vi "IMUread.vi"() -> ()   [LabVIEW 2015]
doc: "The myRIO Project template acquires acceleration data from the onboard accelerometer and displays the changes of acceleration values in a waveform chart."
uses:
  <vilib>/myRIO/Instrument Drivers/Onboard IO/I2C/typedefs/I2C User Configuration.ctl
  <vilib>/myRIO/Instrument Drivers/Onboard IO/I2C/typedefs/I2C Transfer Rate.ctl
  <vilib>/Platform/TimedLoop/XDataNode/timing_clust.ctl
  <vilib>/Platform/TimedLoop/XDataNode/nitl_modes.ctl
  <vilib>/Platform/TimedLoop/XDataNode/wakeup.ctl
  <vilib>/myRIO/Common/Instrument Driver Framework/myRIO v1.0/UART/vis/myRIO v1.0 Close UART.vi
  <vilib>/Utility/error.llb/Error Cluster From Error Code.vi
  <vilib>/myRIO/Common/Instrument Driver Framework/myRIO v1.0/I2C/vis/myRIO v1.0 Configure I2C.vi
  <vilib>/myRIO/Common/Instrument Driver Framework/myRIO v1.0/I2C/vis/myRIO v1.0 Write I2C.vi
  <vilib>/myRIO/Common/Instrument Driver Framework/myRIO v1.0/I2C/vis/myRIO v1.0 Read I2C.vi
  <vilib>/myRIO/Common/Instrument Driver Framework/Utilities/vis/FPGA Ref Manager.vi
  <vilib>/myRIO/Common/Instrument Driver Framework/myRIO v1.0/myRIO v1.0 Reset FPGA.vi
  <vilib>/myRIO/Common/Instrument Driver Framework/myRIO v1.0/IRQ/vis/myRIO v1.0 IRQ Info FGV.vi
  <vilib>/myRIO/Common/Instrument Driver Framework/myRIO v1.0/IRQ/vis/myRIO v1.0 Timer IRQ Info FGV.vi
  <vilib>/myRIO/Common/Instrument Driver Framework/myRIO v1.0/IRQ/vis/myRIO v1.0 ISR Agent.vi
  <vilib>/platform/TimedLoop/XDataNode/XDataNode.xnode
  <vilib>/myRIO/Instrument Drivers/Utilities/Utilities.lvlib
  <vilib>/myRIO/Instrument Drivers/Onboard IO/I2C/I2C.lvlib
  <vilib>/Platform/TimedLoop/XDataNode/XDNodeRunTimeDep.lvlib
panel:
  out "Mag Chart":cluster{dbl, dbl, dbl}(graph)
  out "Acc Chart":cluster{dbl, dbl, dbl}(graph)
  out "Gyro Chart":cluster{dbl, dbl, dbl}(graph)
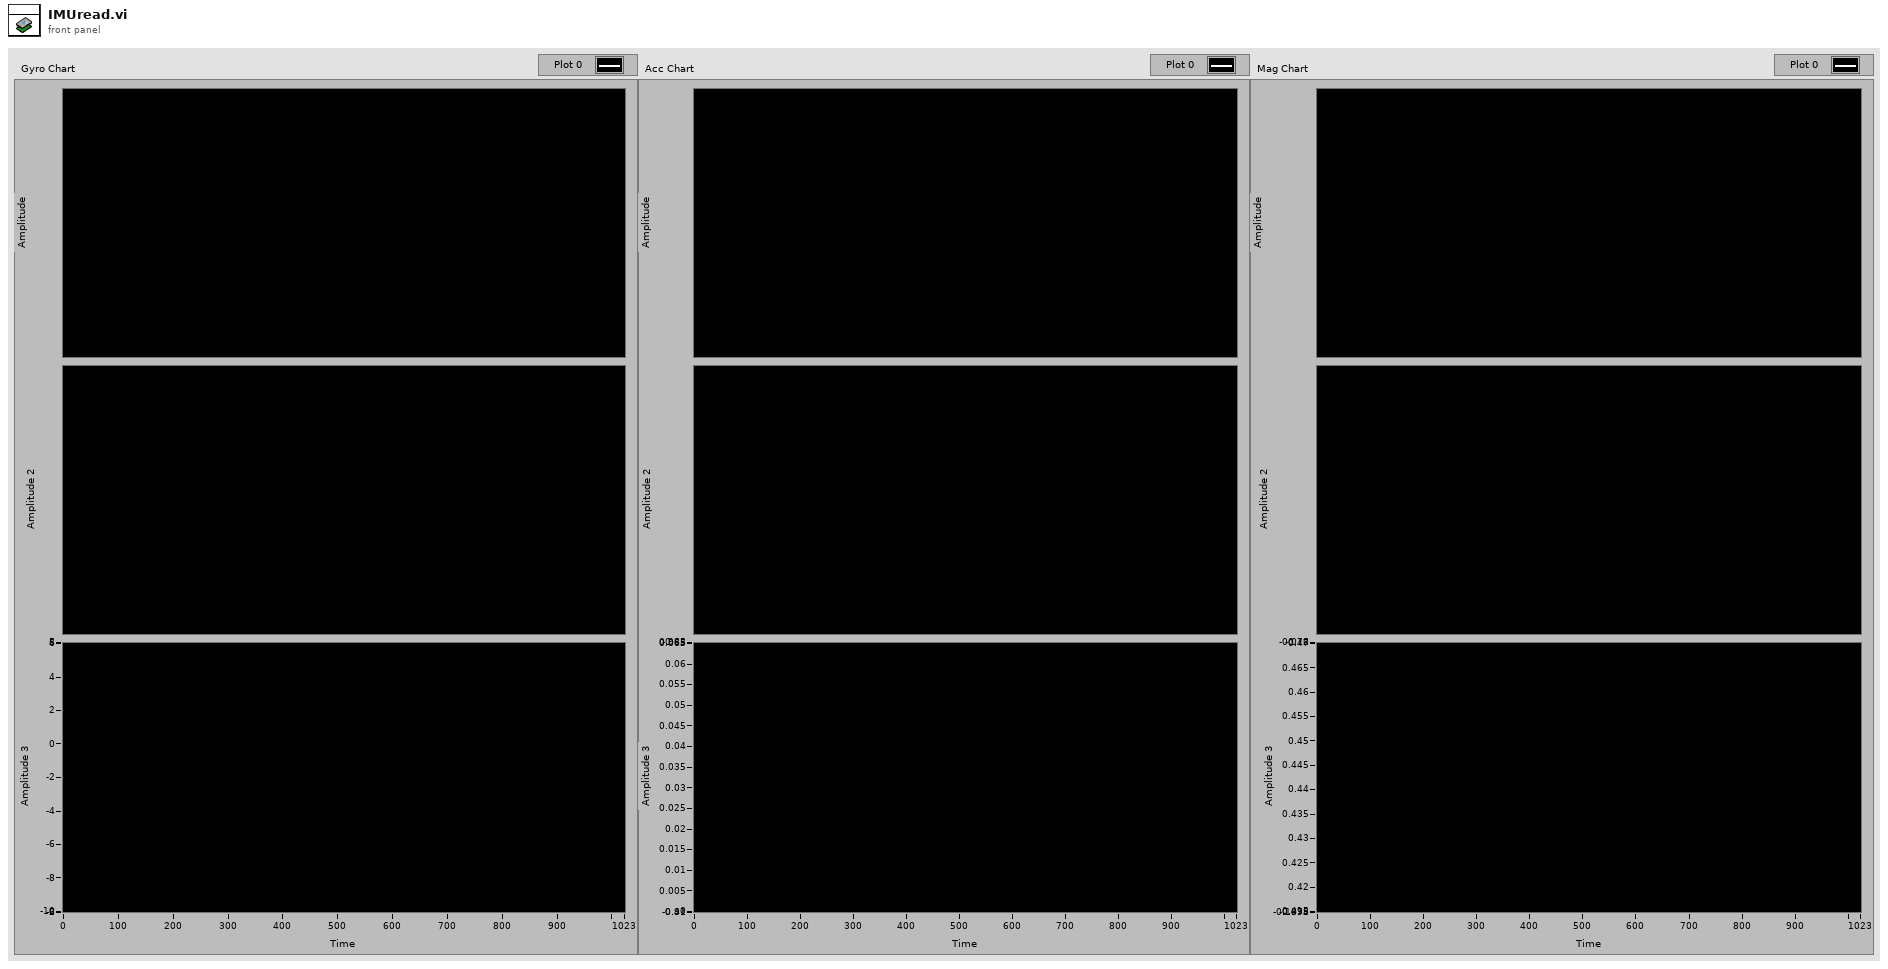
[diagram p1: front panel]
types:
  T1 = typedef "I2C.lvlib/I2C User Configuration.ctl" = cluster{"I2C Transfer Rate":T2}
  T2 = typedef "I2C.lvlib/I2C Transfer Rate.ctl" = enum16{"Standard mode (100 kbps)", "Fast mode (400 kbps)"}
  T3 = typedef "I2C.lvlib/I2C Reference.ctl" = cluster{"myRIO Reference":T4, "I2C Channels Enum":T8, "I2C Configuration":T9}
  T4 = typedef "myRIO Generic Hardware Reference.ctl" = cluster{"myRIO Model":T5, "myRIO Hardware Reference":T6}
  T5 = typedef "Hardware Version Enum.ctl" = enum16{"Unknown", "myRIO-1900", "myRIO-1950", "roboRIO"}
  T6 = typedef "myRIO v1.0 Reference.ctl" = cluster{"Generic FPGA Reference":T7, "Allow multiple opens":bool}
  T7 = typedef "Generic FPGA Reference.ctl" = refnum<k20>
  T8 = typedef "I2C Channels Enum.ctl" = enum16{"Not Connected", "A/I2C", "B/I2C", "I2C/I2C"}
  T9 = typedef "I2C.lvlib/I2C Configuration.ctl" = cluster{"I2C Transfer Rate":T2}
  T10 = typedef "XDNodeRunTimeDep.lvlib/timing_clust.ctl" = cluster{"Expected End [f-1]":u64, "Actual End [f-1]":u64, "Finished Late? [f-1]":bool, "Expected End [i-1]":u64, "Actual End [i-1]":u64, "Finished Late? [i-1]":bool, "Expected Start [i]":u64, "Actual Start [i]":u64, "Expected Start [f]":u64, "Actual Start [f]":u64, "Source Name":string, "Structure Name":string, "Period":i64, "Deadline":i64, "Offset":i64, "Start":i64, "Priority":i32, "Timeout":i32, "Mode":T11, "Wakeup Reason":T12, "Error":errorcluster, "Source Type":string, "Secondary Source Type":string, "Global End Time":u64, "Global Start Time":u64, "Frame Duration":u64, "Iteration Duration":u64, "Assigned CPU":i32, "I/O Scan Engine Mode":u32}
  T11 = typedef "XDNodeRunTimeDep.lvlib/nitl_modes.ctl" = enum32{"No Change", "Process missed periods, maintain original phase", "Discard missed periods, maintain original phase", "Process missed periods, ignore original phase", "Discard missed periods, ignore original phase"}
  T12 = typedef "XDNodeRunTimeDep.lvlib/wakeup.ctl" = enum32{"Normal", "Aborted", "Asynchronous wakeup", "Timing source error", "Timed loop error", "Timeout"}
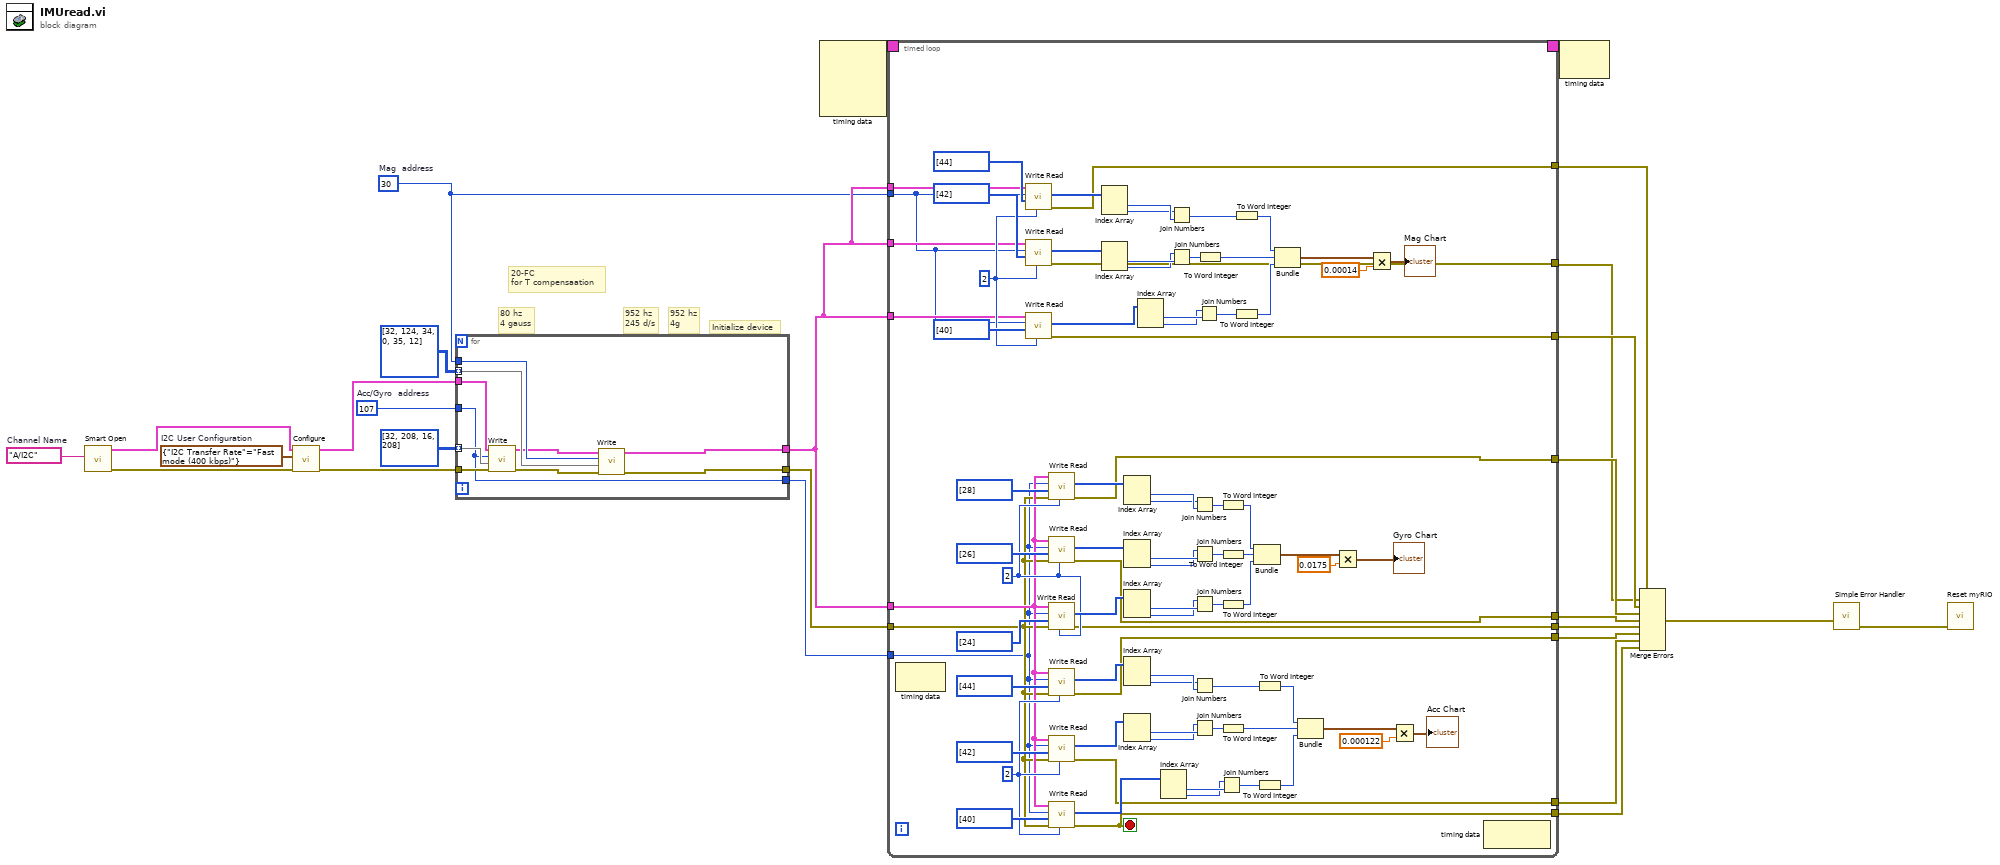
[diagram p0: block diagram]
diagram:
  w2 = u8 30  # Mag  address
  w19 = u8 107  # Acc/Gyro  address
  w22 = T1 {"I2C Transfer Rate"=enum."Fast mode (400 kbps)"}  # I2C User Configuration
  w23 = tag "A/I2C"  # Channel Name
  # "20-FC\nfor T compensaation"
  # "80 hz\n4 gauss"
  # "952 hz\n4g"
  # "952 hz\n245 d/s"
  # "Initialize device"
  n1 = call <vilib>:"Smart Open.vi"("Channel Name"=w23) -> ("error out"=w20:errorcluster, "I2C Ref Out"=w21:T3)  [unwired: 9 in]
  n2 = call <vilib>:"Configure.vi"("error in (no error)"=w20, "I2C User Configuration"=w22, "I2C Ref In"=w21) -> ("error out"=w9:errorcluster, "I2C Ref Out"=w10:T3)  [unwired: 7 in]
  n3 = for {
    tunnel: [w28] -> w7
    tunnel: [w27] -> w3
    tunnel: [w33] -> w14
    tunnel: u8[][] [[32, 208], [16, 208]] ("Bytes to Write") -> [w34] mode=indexing
    tunnel: w10 -> [w36]
    tunnel: w9 -> [w35]
    tunnel: w19 -> [w33]
    tunnel: u8[][] [[32, 124], [34, 0], [35, 12]] ("Bytes to Write") -> [w32] mode=indexing
    tunnel: w2 -> [w31]
    n4 = call <vilib>:"Write.vi"("error in (no error)"=w35, "Bytes to Write"=w34, "Slave Address (7-bit)"=w33, "I2C Ref In"=w36) -> ("error out"=w29:errorcluster, "I2C Ref Out"=w30:T3)  [unwired: 6 in]
    n5 = call <vilib>:"Write.vi"("error in (no error)"=w29, "Bytes to Write"=w32, "Slave Address (7-bit)"=w31, "I2C Ref In"=w30) -> ("error out"=w28:errorcluster, "I2C Ref Out"=w27:T3)  [unwired: 6 in]
  }
  n6 = node-c288() -> (w25:T10)  [unwired: 4 in]
  n7 = timed-loop {
    tunnel: [w109] -> w15
    timing: w25 -> [_]
    timing-out: [_] -> w24
    tunnel: w14 -> [w68]
    tunnel: w7 -> [w72]
    tunnel: w3 -> [w73]
    tunnel: [w103] -> w17
    tunnel: [w102] -> w16
    tunnel: [w71] -> w13
    tunnel: [w70] -> w12
    tunnel: [w69] -> w11
    tunnel: [w43] -> w6
    tunnel: [w42] -> w5
    tunnel: [w41] -> w4
    tunnel: w3 -> [w40]
    tunnel: w3 -> [w39]
    tunnel: w3 -> [w38]
    tunnel: w2 -> [w37]
    stop <- w109 stop-if-true
    w51 = u32 2 ("Byte Count")
    w74 = u32 2 ("Byte Count")
    w95 = u32 2 ("Byte Count")
    n8 = node-c288() -> ()  [unwired: 1 in, 1 out]
    n9 = call <vilib>:"Write Read.vi"("Byte Count"=w51, "Bytes to Write"=u8[] [44], "Slave Address (7-bit)"=w37, "I2C Ref In"=w38) -> ("error out"=w42:errorcluster, "Bytes Read"=w53:u8[])  [unwired: 4 in, 1 out]
    n10 = call <vilib>:"Write Read.vi"("Byte Count"=w51, "Bytes to Write"=u8[] [42], "Slave Address (7-bit)"=w37, "I2C Ref In"=w39) -> ("error out"=w41:errorcluster, "Bytes Read"=w55:u8[])  [unwired: 4 in, 1 out]
    n11 = call <vilib>:"Write Read.vi"("Byte Count"=w51, "Bytes to Write"=u8[] [40], "Slave Address (7-bit)"=w37, "I2C Ref In"=w40) -> ("error out"=w43:errorcluster, "Bytes Read"=w62:u8[])  [unwired: 4 in, 1 out]
    n12 = call <vilib>:"Write Read.vi"("Byte Count"=w74, "error in (no error)"=w72, "Bytes to Write"=u8[] [28], "Slave Address (7-bit)"=w68, "I2C Ref In"=w73) -> ("error out"=w69:errorcluster, "Bytes Read"=w82:u8[])  [unwired: 3 in, 1 out]
    n13 = call <vilib>:"Write Read.vi"("Byte Count"=w74, "error in (no error)"=w72, "Bytes to Write"=u8[] [26], "Slave Address (7-bit)"=w68, "I2C Ref In"=w73) -> ("error out"=w70:errorcluster, "Bytes Read"=w84:u8[])  [unwired: 3 in, 1 out]
    n14 = call <vilib>:"Write Read.vi"("Byte Count"=w74, "error in (no error)"=w72, "Bytes to Write"=u8[] [24], "Slave Address (7-bit)"=w68, "I2C Ref In"=w73) -> ("error out"=w71:errorcluster, "Bytes Read"=w91:u8[])  [unwired: 3 in, 1 out]
    n15 = call <vilib>:"Write Read.vi"("Byte Count"=w95, "error in (no error)"=w72, "Bytes to Write"=u8[] [44], "Slave Address (7-bit)"=w68, "I2C Ref In"=w73) -> ("error out"=w103:errorcluster, "Bytes Read"=w105:u8[])  [unwired: 3 in, 1 out]
    n16 = call <vilib>:"Write Read.vi"("Byte Count"=w95, "error in (no error)"=w72, "Bytes to Write"=u8[] [42], "Slave Address (7-bit)"=w68, "I2C Ref In"=w73) -> ("error out"=w102:errorcluster, "Bytes Read"=w107:u8[])  [unwired: 3 in, 1 out]
    n17 = call <vilib>:"Write Read.vi"("Byte Count"=w95, "error in (no error)"=w72, "Bytes to Write"=u8[] [40], "Slave Address (7-bit)"=w68, "I2C Ref In"=w73) -> ("error out"=w109:errorcluster, "Bytes Read"=w115:u8[])  [unwired: 3 in, 1 out]
    n18 = Index Array "Index Array"(array=w53) -> (element #1=w46:u8, element #2=w45:u8)  [unwired: 2 in]
    n19 = Index Array "Index Array"(array=w55) -> (element #1=w50:u8, element #2=w49:u8)  [unwired: 2 in]
    n20 = Index Array "Index Array"(array=w82) -> (element #1=w80:u8, element #2=w79:u8)  [unwired: 2 in]
    n21 = Index Array "Index Array"(array=w84) -> (element #1=w78:u8, element #2=w77:u8)  [unwired: 2 in]
    n22 = Index Array "Index Array"(array=w91) -> (element #1=w76:u8, element #2=w75:u8)  [unwired: 2 in]
    n23 = Index Array "Index Array"(array=w105) -> (element #1=w101:u8, element #2=w100:u8)  [unwired: 2 in]
    n24 = Index Array "Index Array"(array=w107) -> (element #1=w99:u8, element #2=w98:u8)  [unwired: 2 in]
    n25 = Index Array "Index Array"(array=w62) -> (element #1=w48:u8, element #2=w47:u8)  [unwired: 2 in]
    n26 = Index Array "Index Array"(array=w115) -> (element #1=w97:u8, element #2=w96:u8)  [unwired: 2 in]
    n27 = Join Numbers(hi=w45, lo=w46) -> ((hi.lo)=w65:u16)
    n28 = Join Numbers(hi=w49, lo=w50) -> ((hi.lo)=w64:u16)
    n29 = Join Numbers(hi=w79, lo=w80) -> ((hi.lo)=w94:u16)
    n30 = Join Numbers(hi=w77, lo=w78) -> ((hi.lo)=w93:u16)
    n31 = Join Numbers(hi=w75, lo=w76) -> ((hi.lo)=w92:u16)
    n32 = Join Numbers(hi=w100, lo=w101) -> ((hi.lo)=w118:u16)
    n33 = Join Numbers(hi=w98, lo=w99) -> ((hi.lo)=w117:u16)
    n34 = Join Numbers(hi=w47, lo=w48) -> ((hi.lo)=w63:u16)
    n35 = To Word Integer(number=w64) -> (16bit integer=w58:i16)
    n36 = Join Numbers(hi=w96, lo=w97) -> ((hi.lo)=w116:u16)
    n37 = To Word Integer(number=w94) -> (16bit integer=w88:i16)
    n38 = To Word Integer(number=w93) -> (16bit integer=w87:i16)
    n39 = To Word Integer(number=w92) -> (16bit integer=w86:i16)
    n40 = To Word Integer(number=w117) -> (16bit integer=w111:i16)
    n41 = To Word Integer(number=w65) -> (16bit integer=w59:i16)
    n42 = To Word Integer(number=w63) -> (16bit integer=w57:i16)
    n43 = Bundle "Bundle"(w88, w87, w86) -> (w89:cluster{i16, i16, i16})  [unwired: 1 in]
    n44 = To Word Integer(number=w118) -> (16bit integer=w112:i16)
    n45 = To Word Integer(number=w116) -> (16bit integer=w110:i16)
    n46 = Bundle "Bundle"(w59, w58, w57) -> (w60:cluster{i16, i16, i16})  [unwired: 1 in]
    n47 = Bundle "Bundle"(w112, w111, w110) -> (w113:cluster{i16, i16, i16})  [unwired: 1 in]
    n48 = Multiply(x=w89, y=0.0175) -> (x*y=→"Gyro Chart":cluster{dbl, dbl, dbl})
    n49 = Multiply(x=w60, y=0.00014) -> (x*y=→"Mag Chart":cluster{dbl, dbl, dbl})
    n50 = Multiply(x=w113, y=0.000122) -> (x*y=→"Acc Chart":cluster{dbl, dbl, dbl})
    n51 = node-c288() -> ()  [unwired: 1 in, 1 out]
  }
  n52 = node-c288(w24) -> ()  [unwired: 1 out]
  n53 = Merge Errors(w5, w4, w6, w11, w12, w13, w17, w16, w15) -> (w1:errorcluster)
  n54 = call <vilib>:"Simple Error Handler.vi"("error in (no error)"=w1) -> ("error out"=w26:errorcluster)  [unwired: 4 in, 4 out]
  n55 = call <vilib>:"Reset myRIO.vi"("error in (no error)"=w26) -> ()  [unwired: 10 in, 1 out]
